vi "Springboard Demo - place and adjust arrows.vi"() -> ()   [LabVIEW 2026]
uses:
  <vilib>/Utility/miscctls.llb/LVPositionTypeDef.ctl
  <vilib>/Utility/miscctls.llb/LVBoundsTypeDef.ctl
  Arrow Direction.ctl
panel:
  in  "Size 2":cluster{"Magnitude":dbl, "Angle":dbl} {"Magnitude" scale=5.0..200.0; "Angle" scale=0.0..90.0}
  in  "Arrow Direction":T1
  in  "stop":bool
  in  "Size":T2 {"Width" scale=5.0..100.0; "Height" scale=5.0..100.0}
  in  "Position":T3 {"Left" scale=-100.0..100.0; "Top" scale=-100.0..100.0}
  in  "ACTION":bool
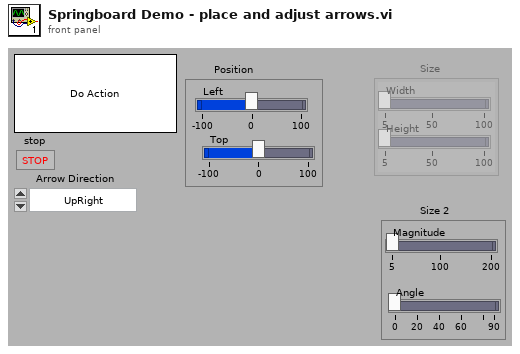
[diagram p1: front panel]
types:
  T1 = typedef "Arrow Direction.ctl" = enum16{"UpRight", "UpLeft", "DownLeft", "DownRight"}
  T2 = typedef "LVBoundsTypeDef.ctl" = cluster{"Width":u32, "Height":u32}
  T3 = typedef "LVPositionTypeDef.ctl" = cluster{"Left":i32, "Top":i32}
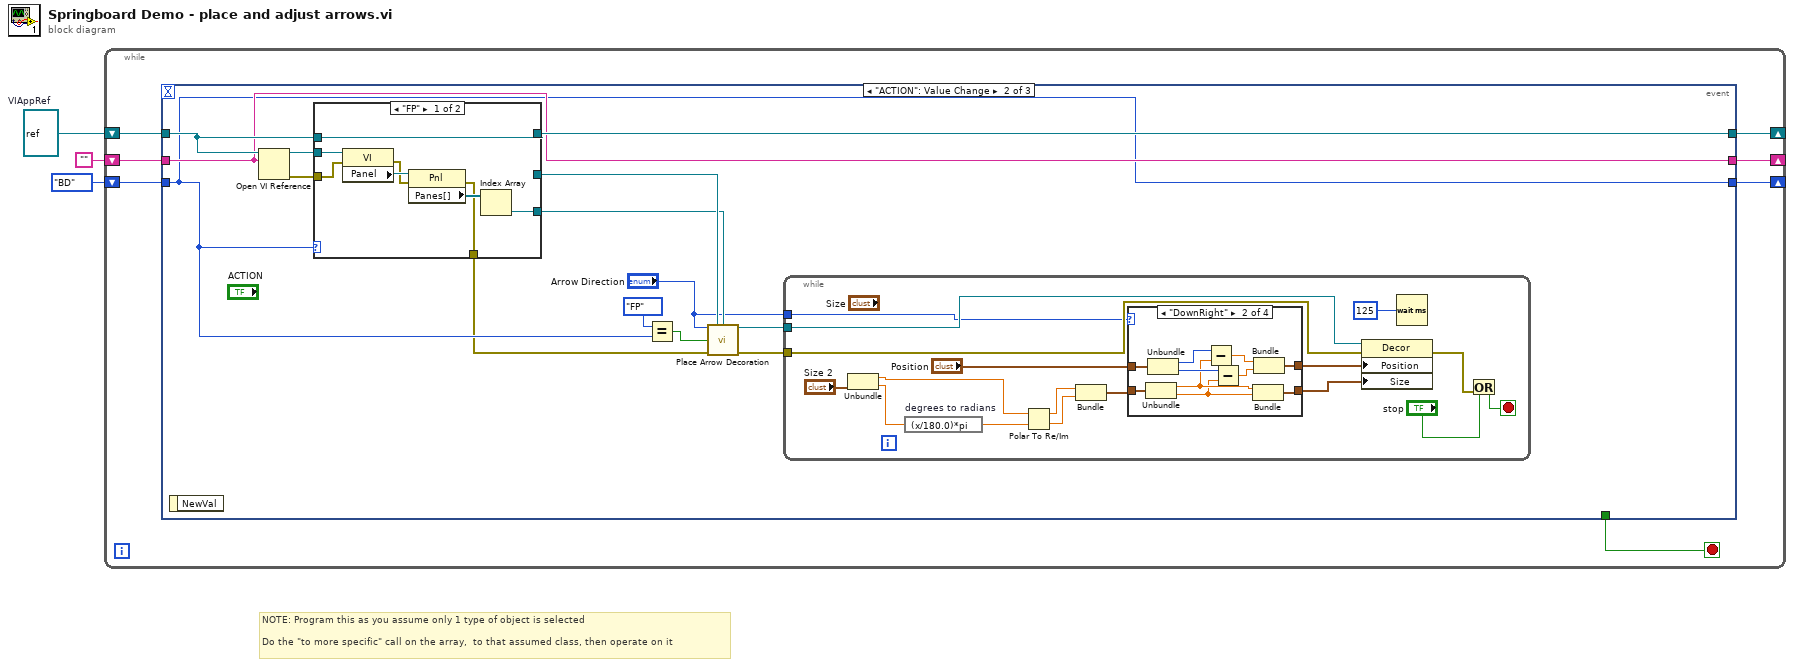
[diagram p0: block diagram]
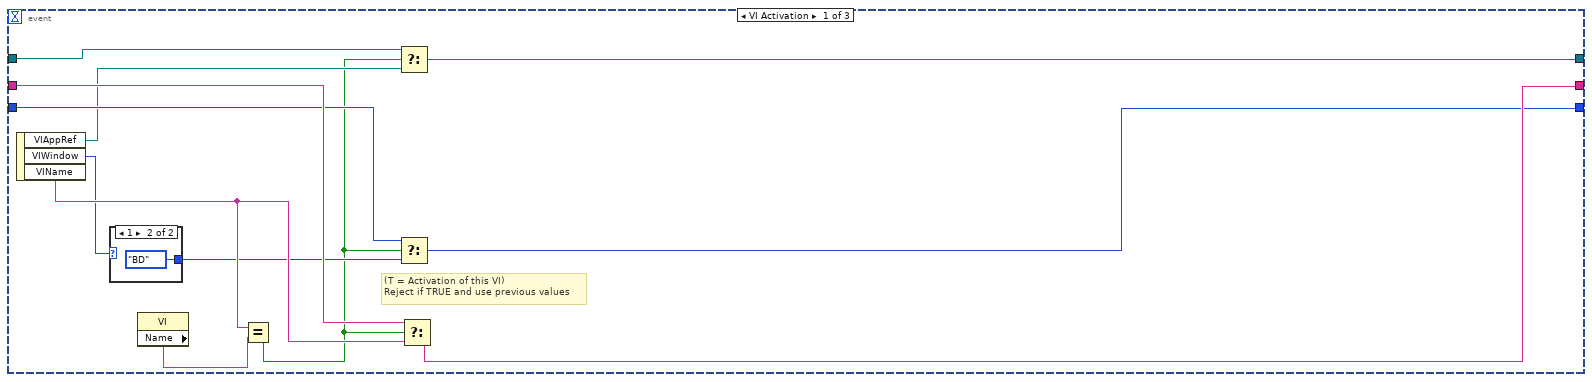
[diagram p2: hidden frame]
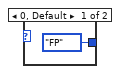
[diagram p3: hidden frame]
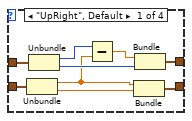
[diagram p4: hidden frame]
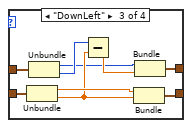
[diagram p5: hidden frame]
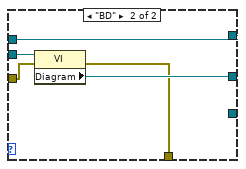
[diagram p7: hidden frame]
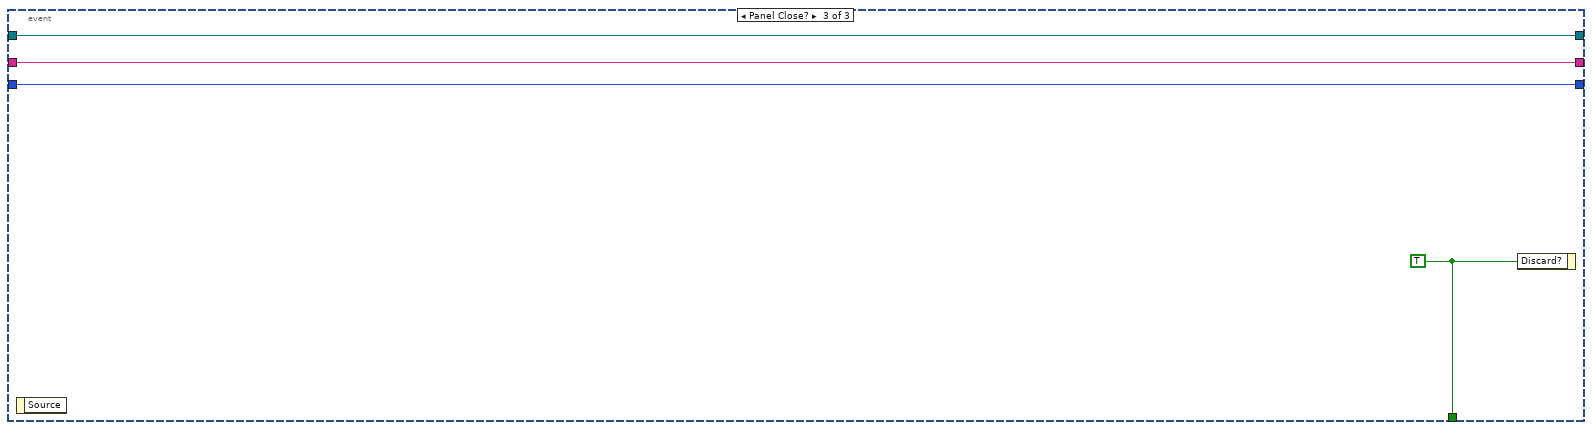
[diagram p8: hidden frame]
diagram:
  w1 = refnum<vi> refnum  # VIAppRef
  # "NOTE: Program this as you assume only 1 type of object is selected\n\nDo the \"to more specific\" call on the array,  to that assumed class, then operate on it"
  n1 = while {
    shift-right: [w10] -> _
    shift-left: "" -> [w9]
    shift-right: [w7] -> _
    shift-left: enum16{"FP", "BD"}."BD" -> [w6]
    shift-right: [w5] -> _
    shift-left: w1 -> [w4]
    stop <- w8 stop-if-true
    n2 = event shown="[1] \"ACTION\": Value Change" {
      selector: _ -> [_ _ _]
      dyn-events: _ -> [_ _ _]
      timeout: _ -> [_ _ _]
      tunnel: [w19 w35 w100] -> w10
      tunnel: w9 -> [w22 w35 w100]
      tunnel: [_ _ w102] -> w8
      tunnel: [w17 w29 w101] -> w7
      tunnel: w6 -> [w18 w29 w101]
      tunnel: [w13 w37 w99] -> w5
      tunnel: w4 -> [w12 w36 w99]
      event VI Activation {
        # "(T = Activation of this VI)\nReject if TRUE and use previous values"
        n3 = event-data() -> ("VIAppRef"=w14:refnum<vi>, "VIWindow"=w16:i32, "VIName"=w20:string)  [unwired: 1 out]
        n4 = case shown="1" w16 {
          tunnel: [enum16{"FP", "BD"}."FP" enum16{"FP", "BD"}."BD"] -> w15
          frame 0, Default {
          }
          frame 1 {
          }
        }
        n5 = property class="VI"() -> ("Name"=w21:string)  [unwired: 2 in, 2 out]
        n6 = Equal?(x=w20, y=w21) -> (x = y?=w11:bool)
        n7 = Select(t=w12, s=w11, f=w14) -> (s? t:f=w13:refnum<vi>)
        n8 = Select(t=w18, s=w11, f=w15) -> (s? t:f=w17:enum16{"FP", "BD"})
        n9 = Select(t=w22, s=w11, f=w20) -> (s? t:f=w19:string)
      }
      event "ACTION": Value Change {
        n10 = event-data() -> ()  [unwired: 2 out]
        n11 = Open VI Reference(application reference (local)=w36, vi path=w35) -> (vi reference=w38:refnum<vi>, error out=w27:errorcluster)  [unwired: 2 in, 2 out]
        n12 = case shown="\"FP\"" w29 {
          tunnel: w38 -> [w93 w98]
          tunnel: [w91 w97] -> w37
          tunnel: w36 -> [w91 w97]
          tunnel: [_ w96] -> w34
          tunnel: [w89 _] -> w33
          tunnel: w27 -> [w88 w95]
          tunnel: [w86 w94] -> w26
          frame "FP" {
            n13 = property class="VI"(reference=w93, error in=w88) -> (error out=w87:errorcluster, "Panel"=w92:refnum<vi>)  [unwired: 1 out]
            n14 = property class="Pnl"(reference=w92, error in=w87) -> (error out=w86:errorcluster, "Panes[]"=w90:refnum<vi>[])  [unwired: 1 out]
            n15 = Index Array(array=w90) -> (element=w89:refnum<vi>)  [unwired: 1 in]
          }
          frame "BD" {
            n16 = property class="VI"(reference=w98, error in=w95) -> (error out=w94:errorcluster, "Diagram"=w96:refnum<vi>)  [unwired: 1 out]
          }
        }
        n17 = Equal?(x=enum16{"FP", "BD"}."FP", y=w29) -> (x = y?=w28:bool)
        n18 = call "Place Arrow Decoration.vi"("Arrow Direction"="Arrow Direction", "Diagram"=w34, "Pane Refnum"=w33, "FP? (T)"=w28, "error in"=w26) -> ("Decor Refnum"=w32:refnum<vi>, "error out"=w31:errorcluster)  [unwired: 9 in]
        n19 = while {
          tunnel: w32 -> [w52]
          tunnel: w31 -> [w51]
          tunnel: "Arrow Direction" -> [w46]
          stop <- w48 stop-if-true
          n20 = Unbundle("Size 2") -> ("Magnitude"=w44:dbl, "Angle"=w43:dbl)
          n21 = expression code="(x/180.0)*pi" "degrees to radians"(w43) -> (w42:dbl)
          n22 = Polar To Re/Im(2:w42, 3:w44) -> (0:w40:dbl, 1:w41:dbl)
          n23 = Bundle(w41, w40) -> (w39:cluster{dbl, dbl})  [unwired: 1 in]
          n24 = case shown="\"DownRight\"" w46 {
            tunnel: [w61 w71 w81 w84] -> w55
            tunnel: [w57 w68 w80 w85] -> w49
            tunnel: w39 -> [w64 w74 w83 w85]
            tunnel: "Position" -> [w63 w73 w82 w84]
            frame "UpRight", Default {
              n25 = Unbundle(w64) -> (w56:dbl, w58:dbl)
              n26 = Unbundle(w63) -> ("Left"=w60:i32, "Top"=w62:i32)
              n27 = Subtract(x=w60, y=w56) -> (x-y=w59:dbl)
              n28 = Bundle(w56, w58) -> (w57:cluster{dbl, dbl})  [unwired: 1 in]
              n29 = Bundle(w59, "Top"=w62) -> (w61:cluster{dbl, "Top":i32})  [unwired: 1 in]
            }
            frame "DownRight" {
              n30 = Unbundle(w74) -> (w67:dbl, w65:dbl)
              n31 = Unbundle(w73) -> ("Left"=w70:i32, "Top"=w72:i32)
              n32 = Subtract(x=w70, y=w67) -> (x-y=w69:dbl)
              n33 = Subtract(x=w72, y=w65) -> (x-y=w66:dbl)
              n34 = Bundle(w67, w65) -> (w68:cluster{dbl, dbl})  [unwired: 1 in]
              n35 = Bundle(w69, w66) -> (w71:cluster{dbl, dbl})  [unwired: 1 in]
            }
            frame "DownLeft" {
              n36 = Unbundle(w83) -> (w79:dbl, w77:dbl)
              n37 = Unbundle(w82) -> ("Left"=w75:i32, "Top"=w78:i32)
              n38 = Subtract(x=w78, y=w77) -> (x-y=w76:dbl)
              n39 = Bundle(w79, w77) -> (w80:cluster{dbl, dbl})  [unwired: 1 in]
              n40 = Bundle("Left"=w75, w76) -> (w81:cluster{"Left":i32, dbl})  [unwired: 1 in]
            }
            frame "UpLeft" {
            }
          }
          n41 = property class="Decor"(reference=w52, error in=w51, "Position"=w55, "Size"=w49) -> (error out=w50:errorcluster)  [unwired: 1 out]
          n42 = Wait (ms)(milliseconds to wait=u32 125) -> ()  [unwired: 1 out]
          n43 = Or(x="stop", y=w50) -> (x .or. y?=w48:bool)
        }
      }
      event Panel Close? {
        w102 = TRUE ("Discard?")
        n44 = event-data() -> ()  [unwired: 2 out]
        n45 = event-data("Discard?"=w102) -> ()  [unwired: 1 in, 1 out]
      }
    }
  }
